vi "DoubleSolenoid_Pulse.vi"(4 "Pass_Through_Time":dbl=-1.0 format="%33.4f", 6 "Solenoid Pulse\nTime\nSeconds":dbl=1.5 format="%#_13g", 9 "Solenoid Demand":bool, 11 "Robot Enabled":bool) -> (3 "Solenoid Cmd":T1)   [LabVIEW 2020]
uses:
  <vilib>/Rock Robotics/WPI/Solenoid/WPI_SolenoidValue.ctl
  <vilib>/Rock Robotics/WPI/ThirdParty/JAS_Junk/TrajLib/Timer_New.vi
  <vilib>/Utility/semaphor.llb/Obtain Semaphore Reference.vi
  <vilib>/Rock Robotics/WPI/ThirdParty/JAS_Junk/TrajLib/Timer_Reset.vi
  <vilib>/Rock Robotics/WPI/ThirdParty/JAS_Junk/TrajLib/Timer_Start.vi
  <vilib>/Rock Robotics/WPI/ThirdParty/JAS_Junk/TrajLib/Timer_HasPeriodPassedOnce.vi
  <vilib>/Rock Robotics/WPI/ThirdParty/JAS_Junk/TrajLib/Timer_Stop.vi
  <vilib>/Rock Robotics/WPI/ThirdParty/JAS_Junk/TrajLib/Trajectory_Library.lvlib
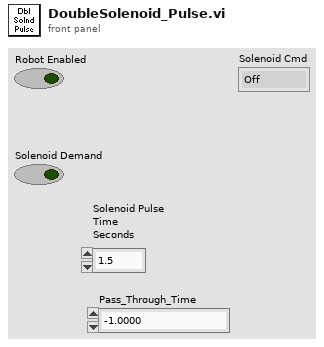
[diagram p1: front panel]
types:
  T1 = typedef "WPI_SolenoidValue.ctl" = enum16{"Off", "On", "Forward", "Reverse"}
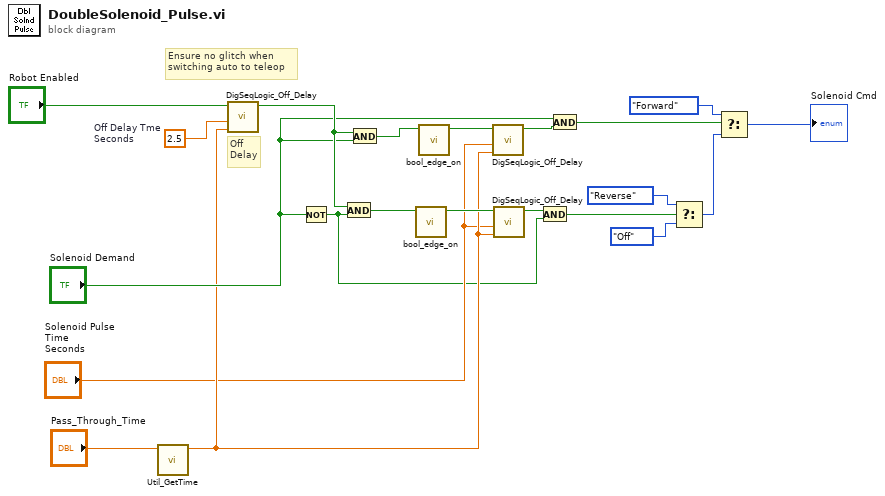
[diagram p0: block diagram]
diagram:
  w16 = 2.5  # Off Delay Tme Seconds
  # "Ensure no glitch when\nswitching auto to teleop"
  # "Off \nDelay"
  n1 = call <vilib>:"Util_GetTime.vi"("Pass_Through_Time"="Pass_Through_Time") -> ("FPGA_Time_Seconds"=w5:dbl)  [unwired: 8 in, 2 out]
  n2 = call <vilib>:"DigSeqLogic_Off_Delay.vi"("Time"=w5, "Delay"=w16, "Input"="Robot Enabled") -> ("Output"=w17:bool)  [unwired: 7 in, 1 out]
  n3 = Not(x="Solenoid Demand") -> (.not. x?=w2:bool)
  n4 = And(x=w17, y=w2) -> (x .and. y?=w7:bool)
  n5 = And(x=w17, y="Solenoid Demand") -> (x .and. y?=w12:bool)
  n6 = call "bool_edge_on.vi"("Input"=w7) -> ("On Edge"=w6:bool)  [unwired: 10 in]
  n7 = call "bool_edge_on.vi"("Input"=w12) -> ("On Edge"=w11:bool)  [unwired: 10 in]
  n8 = call <vilib>:"DigSeqLogic_Off_Delay.vi"("Time"=w5, "Delay"="Solenoid Pulse\nTime\nSeconds", "Input"=w11) -> ("Output"=w10:bool)  [unwired: 7 in, 1 out]
  n9 = call <vilib>:"DigSeqLogic_Off_Delay.vi"("Time"=w5, "Delay"="Solenoid Pulse\nTime\nSeconds", "Input"=w6) -> ("Output"=w3:bool)  [unwired: 7 in, 1 out]
  n10 = And(x=w3, y=w2) -> (x .and. y?=w1:bool)
  n11 = And(x="Solenoid Demand", y=w10) -> (x .and. y?=w8:bool)
  n12 = Select(t=WPI_SolenoidValue."Reverse" ("Value"), s=w1, f=WPI_SolenoidValue."Off" ("Value")) -> (s? t:f=w20:T1)
  n13 = Select(t=WPI_SolenoidValue."Forward" ("Value"), s=w8, f=w20) -> (s? t:f=→"Solenoid Cmd":T1)
